vi "待机状态数据存储写入和切换量程(子VI).vi"   [LabVIEW 2016, in "斯坦道CODMn.lvlib"]
uses:
  <vilib>/ptbypt/NI_PtbyPt.lvlib
types:
  T1 = cluster{"因子编码":u32, "单位":u16, "标样参考值":sgl, "水样数据时间":timestamp, "水样实测值":sgl, "水样数据标识":string, "标样数据时间":timestamp, "标样实测值":sgl, "标样数据标识":string, "空白数据时间":timestamp, "空白实测值":sgl, "空白数据标识":string, "零点核查数据时间":timestamp, "零点核查实测值":sgl, "零点核查数据标识":string, "跨度核查数据时间":timestamp, "跨度核查实测值":sgl, "跨度核查数据标识":string, "加标回收数据时间":timestamp, "加标回收实测值":sgl, "加标回收数据标识":string, "平行样数据时间":timestamp, "平行样实测值":sgl, "平行样数据标识":string}
  T2 = cluster{"时间":timestamp, "测量模式":string, "数据类型":string, "检测值":sgl, "单位":string, "数据标识":string, "因子编码":string, "标样参考值":sgl, "ORP-A":sgl, "ORP-B":sgl, "ORP-K":sgl, "COD滴定值":sgl, "高锰酸钾滴定数":sgl, "温度":sgl, "量程":sgl, "LastTime":timestamp, "序列号:":string, "跨度值":sgl, "高锰酸钾原始滴定数":sgl}
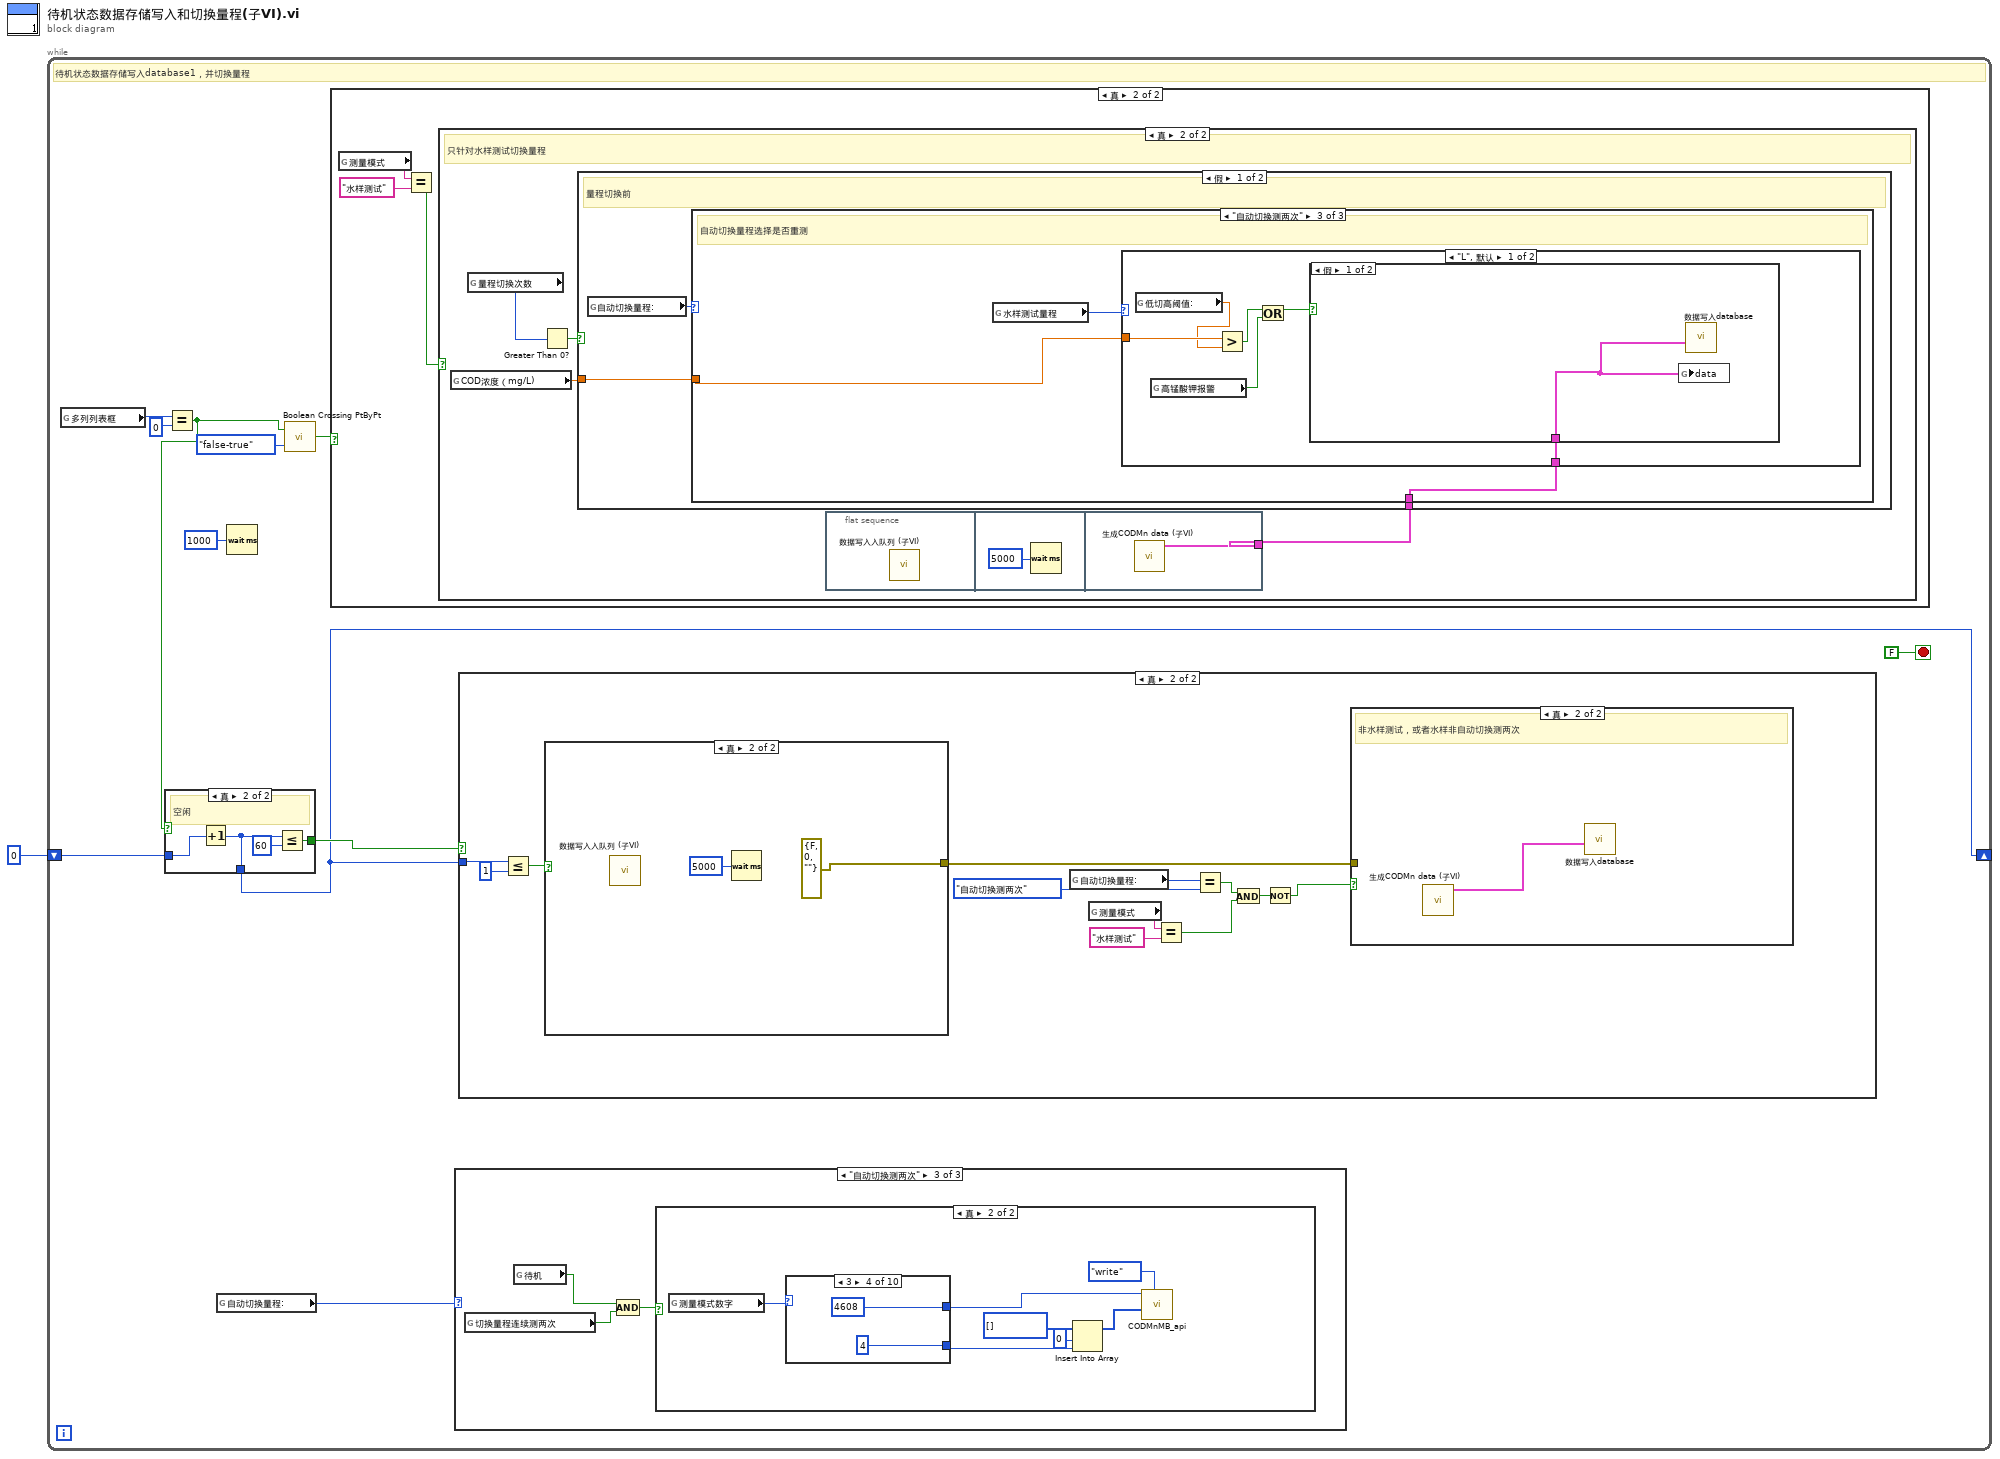
[diagram p0: block diagram]
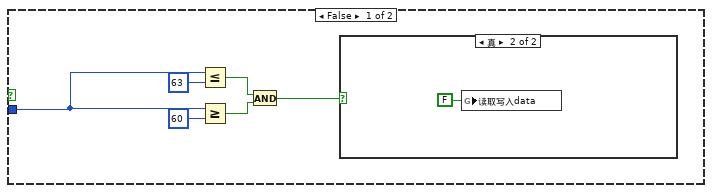
[diagram p2: hidden frame]
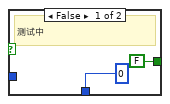
[diagram p6: hidden frame]
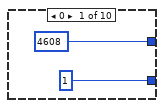
[diagram p10: hidden frame]
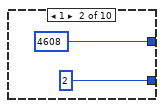
[diagram p11: hidden frame]
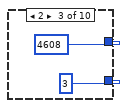
[diagram p12: hidden frame]
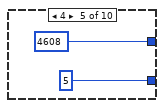
[diagram p13: hidden frame]
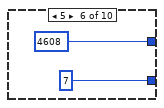
[diagram p14: hidden frame]
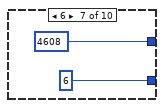
[diagram p15: hidden frame]
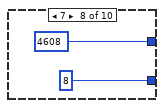
[diagram p16: hidden frame]
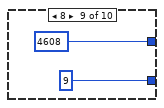
[diagram p17: hidden frame]
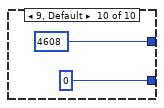
[diagram p18: hidden frame]
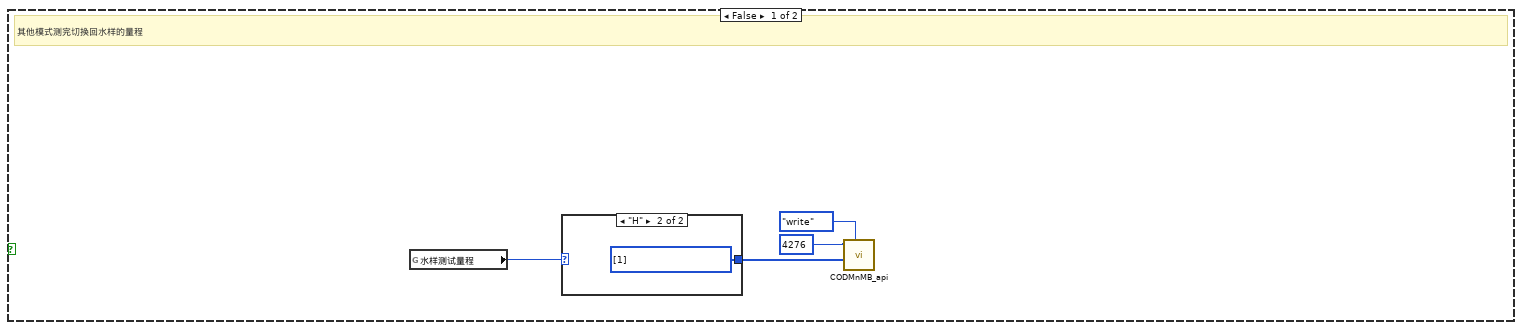
[diagram p20: hidden frame]
diagram:
  n1 = while {
    shift-right: [w2] -> _
    shift-left: 0 ("y") -> [w7]
    stop <- FALSE stop-if-true
    # "待机状态数据存储写入database1，并切换量程"
    n2 = global read "运行时序全局变量.vi" "多列列表框"() -> (w9:i32)
    n3 = Equal?(x=w9, y=0) -> (x = y?=w4:bool)
    n4 = case shown="真" w4 {
      tunnel: w7 -> [_ w39]
      tunnel: [0 w38] -> w2
      tunnel: [FALSE w37] -> w5
      frame False {
        # "测试中"
      }
      frame True {
        # "空闲"
        n5 = Increment(x=w39) -> (x+1=w38:i32)
        n6 = Less Or Equal?(x=w38, y=u32 60) -> (x <= y?=w37:bool)
      }
    }
    n7 = global read "CODMn断电保存全局变量.vi" "自动切换量程:"() -> (w8:enum16{"L", "H", "自动切换测一次", "自动切换测两次"})
    n8 = Wait (ms)(milliseconds to wait=u32 1000 ("等待时间（毫秒）")) -> ()  [unwired: 1 out]
    n9 = call <vilib>:"Boolean Crossing PtByPt.vi"("direction"=enum16{"either", "false-true", "true-false"}."false-true", "input"=w4) -> ("crossing"=w3:bool)  [unwired: 1 in]
    n10 = case shown="真" w3 {
      frame False {
      }
      frame True {
        n11 = global read "COD测量模式全局.vi" "测量模式"() -> (w73:string)
        n12 = Equal?(x=w73, y="水样测试") -> (x = y?=w71:bool)
        n13 = case shown="真" w71 {
          frame False {
            # "其他模式测完切换回水样的量程"
            n14 = global read "CODMn断电保存全局变量.vi" "水样测试量程"() -> (w74:enum16{"L", "H"})
            n15 = case shown="\"H\"" w74 {
              tunnel: [u16[] [0] ("values") u16[] [1] ("values")] -> w75
              frame "L", Default {
              }
              frame "H" {
              }
            }
            n16 = call "CODMnMB_api.vi"("STEP"=enum16{"open", "read", "write", "close"}."write", "values"=w75, "starting address"=u16 4276) -> ()  [unwired: 6 in, 3 out]
          }
          frame True {
            # "只针对水样测试切换量程"
            n17 = global read "COD浓度全局变量.vi" "COD浓度（mg/L)"() -> (w82:dbl)
            n18 = global read "COD内部交互全局.vi" "量程切换次数"() -> (w81:u8)
            n19 = Greater Than 0?(x=w81) -> (x > 0?=w83:bool)
            n20 = case shown="假" w83 {
              tunnel: w80 -> [w86 w136]
              tunnel: w82 -> [w88 _]
              frame False {
                # "量程切换前"
                n21 = global read "CODMn断电保存全局变量.vi" "自动切换量程:"() -> (w87:enum16{"L", "H", "自动切换测一次", "自动切换测两次"})
                n22 = case shown="\"自动切换测两次\"" w87 {
                  tunnel: w88 -> [_ w90 w114]
                  tunnel: w86 -> [_ _ w112]
                  frame "H", Default {
                    # "关闭自动切换量程"
                  }
                  frame "自动切换测一次" {
                    # "自动切换量程选择是否重测"
                    n23 = global read "CODMn断电保存全局变量.vi" "水样测试量程"() -> (w89:enum16{"L", "H"})
                    n24 = global read "COD测量模式全局.vi" "测量模式"() -> (w94:string)
                    n25 = Not Equal?(x=w94, y="水样测试") -> (x != y?=w92:bool)
                    n26 = case shown="真" w92 {
                      tunnel: [w109 w110] -> w91
                      tunnel: w90 -> [w109 _]
                      frame False {
                      }
                      frame True {
                        n27 = global read "CODMn断电保存全局变量.vi" "测量数据区"() -> (w111:T1)
                        n28 = Unbundle By Name(w111) -> ("水样实测值"=w110:sgl)
                      }
                    }
                    n29 = case shown="\"L\", 默认" w89 {
                      tunnel: w91 -> [w98 w104]
                      frame "L", Default {
                        n30 = global read "COD内部交互全局.vi" "高锰酸钾报警"() -> (w95:bool)
                        n31 = global read "CODMn断电保存全局变量.vi" "低切高阈值:"() -> (w96:dbl)
                        n32 = Greater?(x=w98, y=w96) -> (0:w99:bool)
                        n33 = Or(x=w95, y=w99) -> (x .or. y?=w97:bool)
                        n34 = case shown="真" w97 {
                          frame False {
                          }
                          frame True {
                            n35 = call "CODMnMB_api.vi"("STEP"=enum16{"open", "read", "write", "close"}."write", "values"=u16[] [1], "starting address"=u16 4276) -> ()  [unwired: 6 in, 3 out]
                          }
                        }
                      }
                      frame "H" {
                        n36 = global read "CODMn断电保存全局变量.vi" "高切低阈值:"() -> (w103:dbl)
                        n37 = Less?(x=w104, y=w103) -> (x < y?=w105:bool)
                        n38 = case shown="真" w105 {
                          frame False {
                          }
                          frame True {
                            n39 = call "CODMnMB_api.vi"("STEP"=enum16{"open", "read", "write", "close"}."write", "values"=u16[] [0], "starting address"=u16 4276) -> ()  [unwired: 6 in, 3 out]
                          }
                        }
                      }
                    }
                  }
                  frame "自动切换测两次" {
                    # "自动切换量程选择是否重测"
                    n40 = global read "CODMn断电保存全局变量.vi" "水样测试量程"() -> (w113:enum16{"L", "H"})
                    n41 = case shown="\"L\", 默认" w113 {
                      tunnel: w114 -> [w119 w128]
                      tunnel: w112 -> [w115 w126]
                      frame "L", Default {
                        n42 = global read "CODMn断电保存全局变量.vi" "低切高阈值:"() -> (w117:dbl)
                        n43 = global read "COD内部交互全局.vi" "高锰酸钾报警"() -> (w116:bool)
                        n44 = Greater?(x=w119, y=w117) -> (0:w120:bool)
                        n45 = Or(x=w120, y=w116) -> (x .or. y?=w118:bool)
                        n46 = case shown="假" w118 {
                          tunnel: w115 -> [w121 _]
                          frame False {
                            n47 = global write "COD内部交互全局.vi" "data"(w121) -> ()
                            n48 = call "数据写入database.vi"("data输入"=w121) -> ()  [unwired: 10 in, 1 out]
                          }
                          frame True {
                            n49 = global write "COD内部交互全局.vi" "切换量程连续测两次"(TRUE ("切换量程连续测两次")) -> ()
                            n50 = call "CODMnMB_api.vi"("STEP"=enum16{"open", "read", "write", "close"}."write", "values"=u16[] [1], "starting address"=u16 4276) -> ()  [unwired: 6 in, 3 out]
                          }
                        }
                      }
                      frame "H" {
                        n51 = global read "CODMn断电保存全局变量.vi" "高切低阈值:"() -> (w127:dbl)
                        n52 = Less?(x=w128, y=w127) -> (x < y?=w129:bool)
                        n53 = case shown="真" w129 {
                          tunnel: w126 -> [w130 _]
                          frame False {
                            (unwired) "CODMn" ("table")
                            n54 = call "数据写入database.vi"("data输入"=w130) -> ()  [unwired: 10 in, 1 out]
                          }
                          frame True {
                            # "重测第一次不存数据"
                            n55 = call "CODMnMB_api.vi"("STEP"=enum16{"open", "read", "write", "close"}."write", "values"=u16[] [0], "starting address"=u16 4276) -> ()  [unwired: 6 in, 3 out]
                            n56 = global write "COD内部交互全局.vi" "切换量程连续测两次"(TRUE ("切换量程连续测两次")) -> ()
                          }
                        }
                      }
                    }
                  }
                }
              }
              frame True {
                (unwired) "CODMn" ("table")
                # "防止无限切量程"
                n57 = global write "COD内部交互全局.vi" "量程切换次数"(u8 0 ("量程切换次数")) -> ()
                n58 = call "数据写入database.vi"("data输入"=w136) -> ()  [unwired: 10 in, 1 out]
              }
            }
            n59 = flat-sequence {
              tunnel: [w85] -> w80
              frame #0 {
                n60 = call "数据写入入队列 (子VI).vi"() -> ()  [unwired: 12 in]
              }
              frame #1 {
                n61 = Wait (ms)(milliseconds to wait=u32 5000 ("等待时间（毫秒）")) -> ()  [unwired: 1 out]
              }
              frame #2 {
                n62 = call "生成CODMn data (子VI).vi"() -> ("data"=w85:T2)  [unwired: 11 in]
              }
            }
          }
        }
      }
    }
    n63 = case shown="\"自动切换测两次\"" w8 {
      frame "H", Default {
      }
      frame "自动切换测一次" {
      }
      frame "自动切换测两次" {
        n64 = global read "COD内部交互全局.vi" "切换量程连续测两次"() -> (w42:bool)
        n65 = global read "COD内部交互全局.vi" "待机"() -> (w41:bool)
        n66 = Compound Arithmetic op=AND ("复合运算")(w41, w42) -> (w43:bool)
        n67 = case shown="真" w43 {
          frame False {
          }
          frame True {
            n68 = global read "COD内部交互全局.vi" "测量模式数字"() -> (w44:i32)
            n69 = case shown="3" w44 {
              tunnel: [u16 4608 ("address") u16 4608 ("address") u16 4608 ("address") u16 4608 ("address") u16 4608 ("address") u16 4608 ("address") u16 4608 ("address") u16 4608 ("address") u16 4608 ("address") u16 4608 ("address")] -> w45
              tunnel: [u16 1 ("address") u16 2 ("address") u16 3 ("address") u16 4 ("address") u16 5 ("address") u16 7 ("address") u16 6 ("address") u16 8 ("address") u16 9 ("address") u16 0 ("address")] -> w50
              frame 0 {
              }
              frame 1 {
              }
              frame 2 {
              }
              frame 3 {
              }
              frame 4 {
              }
              frame 5 {
              }
              frame 6 {
              }
              frame 7 {
              }
              frame 8 {
              }
              frame 9, Default {
              }
            }
            n70 = Insert Into Array(array=u16[] [] ("values"), index=0 ("索引"), new element=w50) -> (w46:u16[])
            n71 = call "CODMnMB_api.vi"("STEP"=enum16{"open", "read", "write", "close"}."write", "values"=w46, "starting address"=w45) -> ()  [unwired: 6 in, 3 out]
          }
        }
      }
    }
    n72 = case shown="真" w5 {
      tunnel: w2 -> [w15 w31]
      frame False {
        n73 = Less Or Equal?(x=w15, y=63) -> (x <= y?=w18:bool)
        n74 = Greater Or Equal?(x=w15, y=60) -> (x >= y?=w17:bool)
        n75 = And(x=w18, y=w17) -> (x .and. y?=w13:bool)
        n76 = case shown="真" w13 {
          frame False {
          }
          frame True {
            n77 = global write "COD内部交互全局.vi" "读取写入data"(FALSE ("读取写入data")) -> ()
          }
        }
      }
      frame True {
        n78 = Less Or Equal?(x=w31, y=1) -> (x <= y?=w29:bool)
        n79 = case shown="真" w29 {
          tunnel: [_ errorcluster {"status"=FALSE, "code"=0, "source"=""} ("错误常量")] -> w28
          frame False {
          }
          frame True {
            n80 = call "数据写入入队列 (子VI).vi"() -> ()  [unwired: 12 in]
            n81 = Wait (ms)(milliseconds to wait=u32 5000 ("等待时间（毫秒）")) -> ()  [unwired: 1 out]
          }
        }
        n82 = global read "CODMn断电保存全局变量.vi" "自动切换量程:"() -> (w25:enum16{"L", "H", "自动切换测一次", "自动切换测两次"})
        n83 = global read "COD测量模式全局.vi" "测量模式"() -> (w26:string)
        n84 = Equal?(x=w26, y="水样测试") -> (x = y?=w22:bool)
        n85 = Equal?(x=w25, y=enum16{"L", "H", "自动切换测一次", "自动切换测两次"}."自动切换测两次") -> (x = y?=w23:bool)
        n86 = And(x=w23, y=w22) -> (x .and. y?=w21:bool)
        n87 = Not(x=w21) -> (.not. x?=w20:bool)
        n88 = case shown="真" w20 {
          tunnel: w28 -> [_ _]
          frame False {
            # "自动切换测两次并且为水样测试"
          }
          frame True {
            # "非水样测试，或者水样非自动切换测两次"
            n89 = call "生成CODMn data (子VI).vi"() -> ("data"=w34:T2)  [unwired: 11 in]
            n90 = call "数据写入database.vi"("data输入"=w34) -> ()  [unwired: 10 in, 1 out]
          }
        }
      }
    }
  }
